vi "counter.vi"() -> ()   [LabVIEW 2015]
uses:
  <vilib>/myRIO/Instrument Drivers/Onboard IO/DIO/typedefs/DIO Reference.ctl
  <vilib>/myRIO/Common/Instrument Driver Framework/Utilities/typedefs/myRIO Generic Hardware Reference.ctl
  <vilib>/myRIO/Common/Instrument Driver Framework/Utilities/typedefs/Hardware Version Enum.ctl
  <vilib>/myRIO/Common/Instrument Driver Framework/Utilities/typedefs/myRIO v1.0 Reference.ctl
  <vilib>/myRIO/Common/Instrument Driver Framework/Utilities/typedefs/Generic FPGA Reference.ctl
  <vilib>/myRIO/Common/Instrument Driver Framework/myRIO v1.0/DIO/typedefs/DIO Channels List.ctl
  <vilib>/myRIO/Common/Instrument Driver Framework/myRIO v1.0/DIO/typedefs/DIO Channels Enum.ctl
  <vilib>/userDefined/High Color/nirio_resource_hc.ctl
  <vilib>/myRIO/Common/Instrument Driver Framework/Utilities/vis/Is FPGA Ref Available.vi
  <vilib>/myRIO/Common/Instrument Driver Framework/myRIO v1.0/DIO/vis/myRIO v1.1 Open DIO.vi
  <vilib>/myRIO/Instrument Drivers/Onboard IO/DIO/vis/Write.vi
  <vilib>/myRIO/Common/Instrument Driver Framework/Utilities/vis/Validate Channels.vi
  <vilib>/myRIO/Common/Instrument Driver Framework/myRIO v1.0/DIO/vis/myRIO v1.0 Reserve DIO.vi
  <vilib>/myRIO/Common/Instrument Driver Framework/myRIO v1.0/Resource Manager/vis/myRIO v1.0 Reserve Channel List.vi
  <vilib>/myRIO/Common/Instrument Driver Framework/myRIO v1.0/DIO/vis/myRIO v1.0 Build MUX Configuration DIO.vi
  <vilib>/myRIO/Common/Instrument Driver Framework/myRIO v1.0/Resource Manager/vis/myRIO v1.0 Reserve Channel.vi
  <vilib>/myRIO/Common/Instrument Driver Framework/myRIO v1.0/Resource Manager/vis/myRIO v1.0 Unreserve Channel.vi
  <vilib>/myRIO/Common/Instrument Driver Framework/myRIO v1.0/Resource Manager/vis/myRIO v1.0 Create Configuration List.vi
  <vilib>/myRIO/Common/Instrument Driver Framework/myRIO v1.0/Resource Manager/vis/myRIO v1.0 Build Mutex Name.vi
  <vilib>/Utility/VariantDataType/GetNumericInfo.vi
  <vilib>/Utility/error.llb/Error Cluster From Error Code.vi
  <vilib>/myRIO/Common/Instrument Driver Framework/myRIO v1.0/myRIO v1.1 Open.vi
  <vilib>/myRIO/Common/Instrument Driver Framework/Utilities/vis/IO Manager.vi
  <vilib>/myRIO/Common/Instrument Driver Framework/Utilities/vis/Configuration Manager.vi
  <vilib>/myRIO/Common/Instrument Driver Framework/myRIO v1.0/Resource Manager/vis/myRIO v1.0 Configure IO.vi
  <vilib>/myRIO/Common/Instrument Driver Framework/myRIO v1.0/myRIO v1.0 Close.vi
  <vilib>/myRIO/Common/Instrument Driver Framework/myRIO v1.0/DIO/vis/myRIO v1.0 Write DIO.vi
  <vilib>/myRIO/Express VI/Onboard Devices/LED/LED Express VI.xnode
  <vilib>/myRIO/Instrument Drivers/Onboard IO/DIO/vis/myRIO DIO Open.xnode
  <vilib>/myRIO/Instrument Drivers/Onboard IO/DIO/DIO.lvlib
panel:
  out "C-BINARY":i16[](array[numeric])
  in  "SELECTOR":bool
  out "C HEXA":string
  out "LED3":bool
  out "LED2":bool
  out "LED1":bool
  out "LED0":bool
  out "C DEC":u32
  in  "speed (mSec)":u32 caption="SPEED"
  # "LSB"
  # "MSB"
  # "LSB"
  # "MSB"
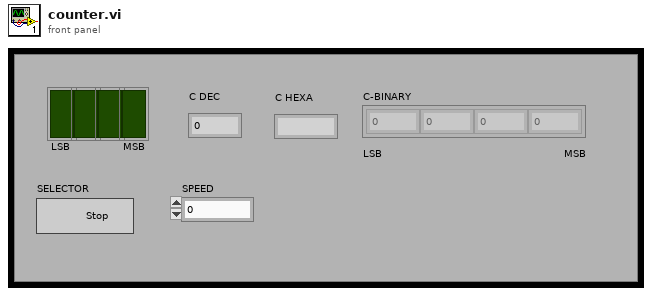
[diagram p1: front panel]
types:
  T1 = typedef "DIO.lvlib/DIO Reference.ctl" = cluster{"myRIO Reference":T2, "DIO Channels List":T6}
  T2 = typedef "myRIO Generic Hardware Reference.ctl" = cluster{"myRIO Model":T3, "myRIO Hardware Reference":T4}
  T3 = typedef "Hardware Version Enum.ctl" = enum16{"Unknown", "myRIO-1900", "myRIO-1950", "roboRIO"}
  T4 = typedef "myRIO v1.0 Reference.ctl" = cluster{"Generic FPGA Reference":T5, "Allow multiple opens":bool}
  T5 = typedef "Generic FPGA Reference.ctl" = refnum<k20>
  T6 = typedef "DIO Channels List.ctl" = T7[]
  T7 = typedef "DIO Channels Enum.ctl" = enum16{"Not Connected", "C/DIO0", "C/DIO1", "C/DIO2", "C/DIO3", "C/DIO4", "C/DIO5", "C/DIO6", "C/DIO7", "A/DIO0", "A/DIO1", "A/DIO2", "A/DIO3", "A/DIO4", "A/DIO5", "A/DIO6", "A/DIO7", "A/DIO8", "A/DIO9", "A/DIO10", "A/DIO11", "A/DIO12", "A/DIO13", "A/DIO14", "A/DIO15", "B/DIO0", "B/DIO1", "B/DIO2", "B/DIO3", "B/DIO4", "B/DIO5", "B/DIO6", "B/DIO7", "B/DIO8", "B/DIO9", "B/DIO10", "B/DIO11", "B/DIO12", "B/DIO13", "B/DIO14", "B/DIO15", "LED0", "LED1", "LED2", "LED3", "Button0", "DIO/DIO0", "DIO/DIO1", "DIO/DIO2", "DIO/DIO3", "DIO/DIO4", "DIO/DIO5", "DIO/DIO6", "DIO/DIO7", "DIO/DIO8", "DIO/DIO9", "SPI/CS0", "SPI/CS1", "SPI/CS2", "SPI/CS3", "LED RADIO (Green)", "LED RADIO (Red)", "LED COMM (Green)", "LED COMM (Red)", "LED MODE (Green)", "LED MODE (Red)"}
  T8 = typedef "nirio_resource_hc.ctl" = tag
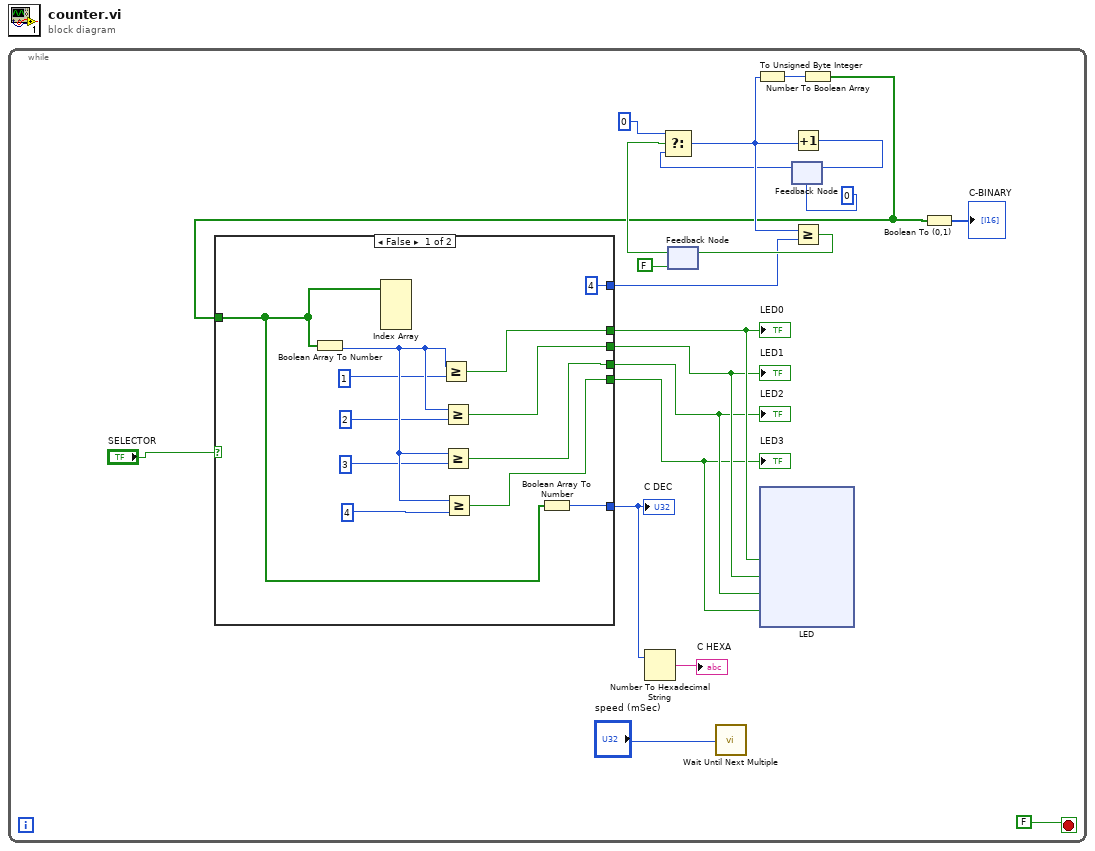
[diagram p0: block diagram]
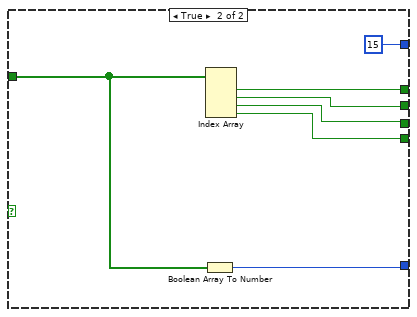
[diagram p2: hidden frame]
diagram:
  n1 = while {
    stop <- FALSE stop-if-true
    n2 = feedback #1(FALSE) -> (w12:bool)
    n3 = call "Wait Until Next Multiple"("Count(mSec)"="speed (mSec)") -> ()  [unwired: 1 out]
    n4 = feedback #2(0) -> (w1:i32)
    n5 = Select(t=0 ("f"), s=w12, f=w1) -> (s? t:f=w7:i32)
    n6 = To Unsigned Byte Integer(number=w7) -> (unsigned 8bit integer=w8:u8)
    n7 = Increment(x=w7) -> (x+1=w9:i32)
    n8 = feedback-in #2(w9) -> ()
    n9 = Number To Boolean Array(number=w8) -> (Boolean array=w3:bool[])
    n10 = case shown="False" "SELECTOR" {
      tunnel: [w65 w78] -> w16
      tunnel: w3 -> [w66 w77]
      tunnel: [w64 w76] -> w21
      tunnel: [w63 w75] -> w20
      tunnel: [w62 w74] -> w19
      tunnel: [w61 w73] -> w18
      tunnel: [4 15] -> w5
      frame False {
        n11 = Boolean Array To Number(Boolean array=w66) -> (number=w71:u32)
        n12 = Index Array(array=w66) -> ()  [unwired: 4 in, 4 out]
        n13 = Greater Or Equal?(x=w71, y=u32 1) -> (x >= y?=w64:bool)
        n14 = Greater Or Equal?(x=w71, y=u32 2) -> (x >= y?=w63:bool)
        n15 = Greater Or Equal?(x=w71, y=u32 3) -> (x >= y?=w62:bool)
        n16 = Greater Or Equal?(x=w71, y=u32 4) -> (x >= y?=w61:bool)
        n17 = Boolean Array To Number(Boolean array=w66) -> (number=w65:u32)
      }
      frame True {
        n18 = Boolean Array To Number(Boolean array=w77) -> (number=w78:u32)
        n19 = Index Array(array=w77) -> (element #1=w76:bool, element #2=w75:bool, element #3=w74:bool, element #4=w73:bool)  [unwired: 4 in]
      }
    }
    "LED0" <- w21
    "LED1" <- w20
    "LED2" <- w19
    "LED3" <- w18
    "C DEC" <- w16
    n20 = Number To Hexadecimal String(2:w16) -> (0:→"C HEXA":string)  [unwired: 1 in]
    n21 = xnode "LED"("LED0"=w21, "LED1"=w20, "LED2"=w19, "LED3"=w18) -> ()  [unwired: 1 in, 1 out]
    n22 = Greater Or Equal?(x=w7, y=w5) -> (x >= y?=w6:bool)
    n23 = feedback-in #1(w6) -> ()
    n24 = Boolean To (0,1)(Boolean=w3) -> (0, 1=→"C-BINARY":i16[])
  }
